vi "Assert N Custom Devices.vi"(8 "error in (no error)":errorcluster, 9 "number of custom devices":i32, 10 "Target in":refnum<k24>, 11 "Test Case in":refnum<class "Scripting API Test Case.lvclass">) -> (0 "error out":errorcluster, 2 "Target out":refnum<k24>, 3 "Test Case out":refnum<class "Scripting API Test Case.lvclass">)   [LabVIEW 2015, in "Scripting API Test Case.lvclass"]
uses:
  Scripting API Test Case.lvclass
  NationalInstruments.VeriStand.SystemDefinitionAPI
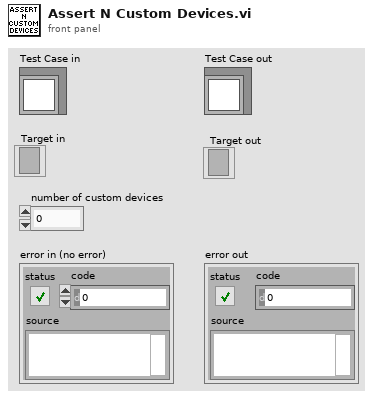
[diagram p1: front panel]
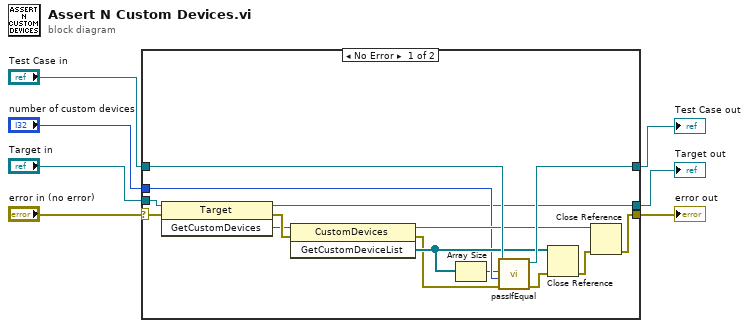
[diagram p0: block diagram]
diagram:
  n1 = case shown="No Error" "error in (no error)" {
    selector: "error in (no error)" -> [w22 w25]
    tunnel: [w21 w25] -> w6
    tunnel: [w20 w24] -> w5
    tunnel: "Test Case in" -> [w19 w24]
    tunnel: "number of custom devices" -> [w13 _]
    tunnel: "Target in" -> [w9 w23]
    tunnel: [w8 w23] -> w1
    frame No Error {
      n2 = invoke class="Target" method="GetCustomDevices"(reference=w9, error in=w22) -> (reference out=w8:refnum<k24>, error out=w11:errorcluster, "GetCustomDevices"=w10:refnum<k24>)  [unwired: 1 in]
      n3 = invoke class="CustomDevices" method="GetCustomDeviceList"(reference=w10, error in=w11) -> (reference out=w18:refnum<k24>, error out=w15:errorcluster, "GetCustomDeviceList"=w16:refnum<k24>[])  [unwired: 1 in]
      n4 = Array Size(array=w16) -> (size(s)=w12:i32)
      n5 = call-dynamic "passIfEqual.vi"("error in (no error)"=w15, "y"=w13, "x"=w12, "TestCase in"=w19) -> ("error out"=w14:errorcluster, "TestCase out"=w20:refnum<class "Scripting API Test Case.lvclass">)  [unwired: 6 in]
      n6 = Close Reference(reference=w16, error in (no error)=w14) -> (error out=w17:errorcluster)
      n7 = Close Reference(reference=w18, error in (no error)=w17) -> (error out=w21:errorcluster)
    }
    frame Error {
    }
  }
  "error out" <- w6
  "Test Case out" <- w5
  "Target out" <- w1
